vi "D-O Module (Main) 2nd.vi"(7 "Name of Parent Panel":string="Main.vi", 9 "New Center Coords":T1={"Horizontal"=470, "Vertical"=200}, 10 "Config":variant, 11 "Main UI Message Queue":refnum<queue>) -> ()   [LabVIEW 2018, in "D-O Module.lvlib"]
uses:
  D-O Module.lvlib
  support/Message Queue/Message Queue.lvlib
  support/Support Library.lvlib
  support/Message Queue/Enqueue Message (Single).vi
  support/Command Log VIs/Command Logging.lvlib
  controls/UI State.ctl
  Sequencing/Squence Update Cluster.ctl
  Sequencing/Sequencing Library.lvlib
  Measure Instrument/State Enum.ctl
  Measure Instrument/Feed Module Engine.lvlib
  support/User Event - Stop/User Event - Stop.lvlib
  D-O Settings Dialog.vi
  <vilib>/Utility/error.llb/Error Cluster From Error Code.vi
  <vilib>/ErrorRing/Error Ring.xnode
  D-O Module Display.ctl
  VICI Electronic Actuator/VICI Electronic Actuator Settings.ctl
  DIO Valve/VICI Electronic Actuator.lvlib
  D-O Device Settings Cluster.ctl
  D-O Module Settings Cluster.ctl
  Valve Clusters.ctl
  <vilib>/Utility/miscctls.llb/LVPoint32TypeDef.ctl
  D-O Module Config Cluster.ctl
  D-O Module State Cluster.ctl
  controls/UI Data.ctl
  Measure Instrument/D-O Module Engine.lvlib
  support/Message Queue/Message Cluster.ctl
panel:
  out "Sequence Started":bool
  out "ScanCode":i16
  in  "Settings Button":bool
  in  "Exit":bool
  out "Ring":u16(ring)=2
  out "Status":string
  out "Log File path":path
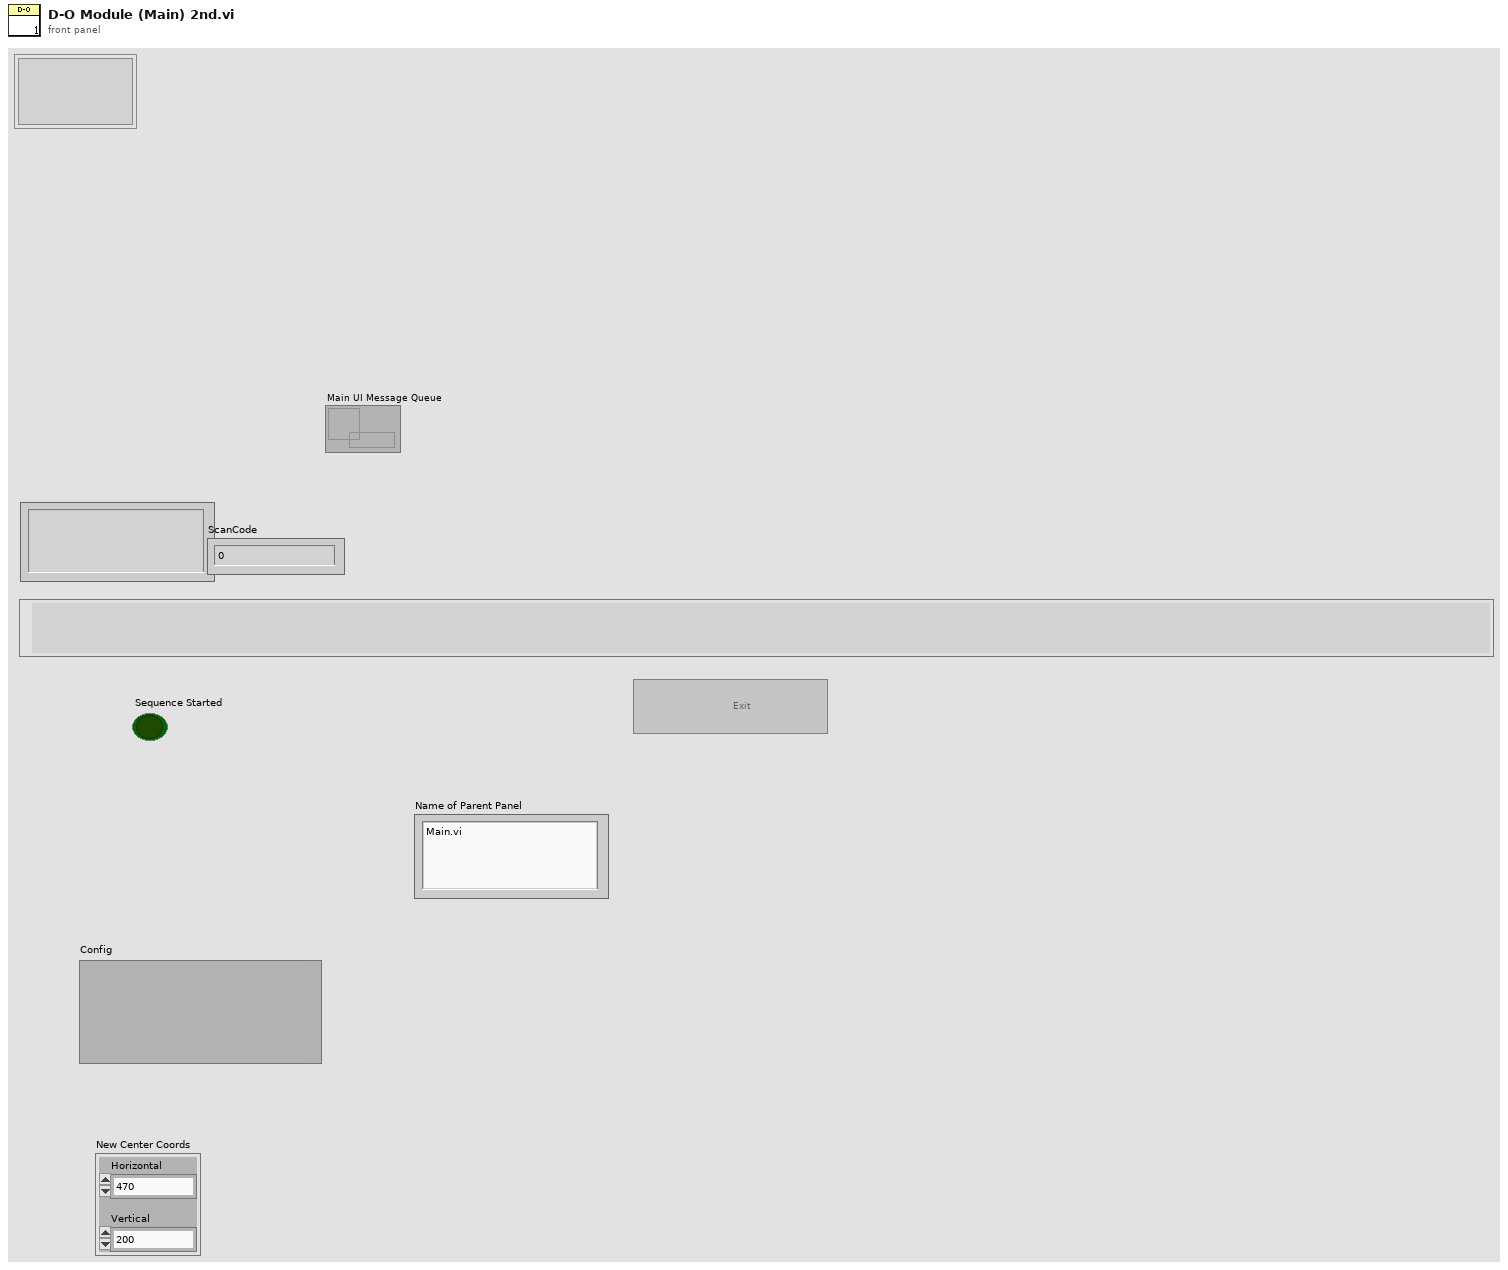
[diagram p1: front panel]
types:
  T1 = typedef "LVPoint32TypeDef.ctl" = cluster{"Horizontal":i32, "Vertical":i32}
  T2 = typedef "UI Data.ctl" = cluster{"Start Ref":refnum<vi>, "Trigger Ref":refnum<vi>, "Stop Ref":refnum<vi>, "Settings Ref":refnum<vi>, "Status Ref":refnum<vi>, "Exit Ref":refnum<vi>, "Data Ref":refnum<vi>}
  T3 = typedef "D-O Module.lvlib/D-O Module State Cluster.ctl" = cluster{"D-O Module Config":T4, "State":T9, "Start Time":timestamp, "Current Time":timestamp, "First Iteration":bool, "Data":cluster{"Valve State":T6}, "Process Name":string, "Queue Name":string, "Program On?":bool}
  T4 = typedef "D-O Module.lvlib/D-O Module Config Cluster.ctl" = cluster{"GUID":string, "Drop Coords":T1, "Process Name":string, "Queue Name":string, "Settings":T5, "Load Count":i32}
  T5 = typedef "D-O Module.lvlib/Valve Clusters.ctl" = cluster{"Valve Settings":T6, "Valve Type":enum16{"Default", "Digital Output Valve", "VICI Electronic Actuator"}, "Time On (Sec)":dbl, "Time Off (Sec)":dbl, "Run?":bool}
  T6 = typedef "D-O Module.lvlib/D-O Module Settings Cluster.ctl" = cluster{"D-O Settings":T7, "VICI Electronic Actuator":T8}
  T7 = typedef "D-O Module.lvlib/D-O Device Settings Cluster.ctl" = cluster{"DAQmx Task Name":refnum<k21>, "Output Channel":u16, "Output Channel Names":string[]}
  T8 = typedef "VICI Electronic Actuator.lvlib/VICI Electronic Actuator Settings.ctl" = cluster{"VISA resource name":refnum<visa-resource-name>, "Mode":enum16{"Two Positions With Stops", "Two Positions Without Stops", "Mutiposition"}, "Simulated":bool}
  T9 = typedef "Feed Module.lvlib/Feed Module Engine.lvlib/State Enum.ctl" = enum16{"Measuring", "Idle", "Paused"}
  T10 = typedef "UI State.ctl" = enum16{"Idle", "Acquiring and Logging", "Waiting for Exit", "Waiting for Exit (Acq Stopped)", "Waiting for Exit (Log Stopped)", "Waiting for Stop", "Waiting for Stop (Acq Stopped)", "Waiting for Stop (Log Stopped)"}
  T11 = typedef "D-O Module.lvlib/All Message Queues.ctl" = cluster{"Engine":refnum<queue>, "D-O UI":refnum<queue>, "D-O Engine":refnum<queue>, "D-O Display":refnum<queue>}
  T12 = typedef "Sequencing Library.lvlib/Squence Update Cluster.ctl" = cluster{"Auto?":bool, "Manual Entry":dbl, "Setpoint":dbl}
  T13 = enum8{"Enabled", "Disabled", "Disabled and Grayed Out"}
  T14 = typedef "D-O Module.lvlib/D-O Module Display.ctl" = cluster{"D-O State ":u16, "Cycle Period":dbl}
  T15 = cluster{"Shift":bool, "Ctrl":bool, "Alt":bool, "Cmd":bool, "Opt":bool}
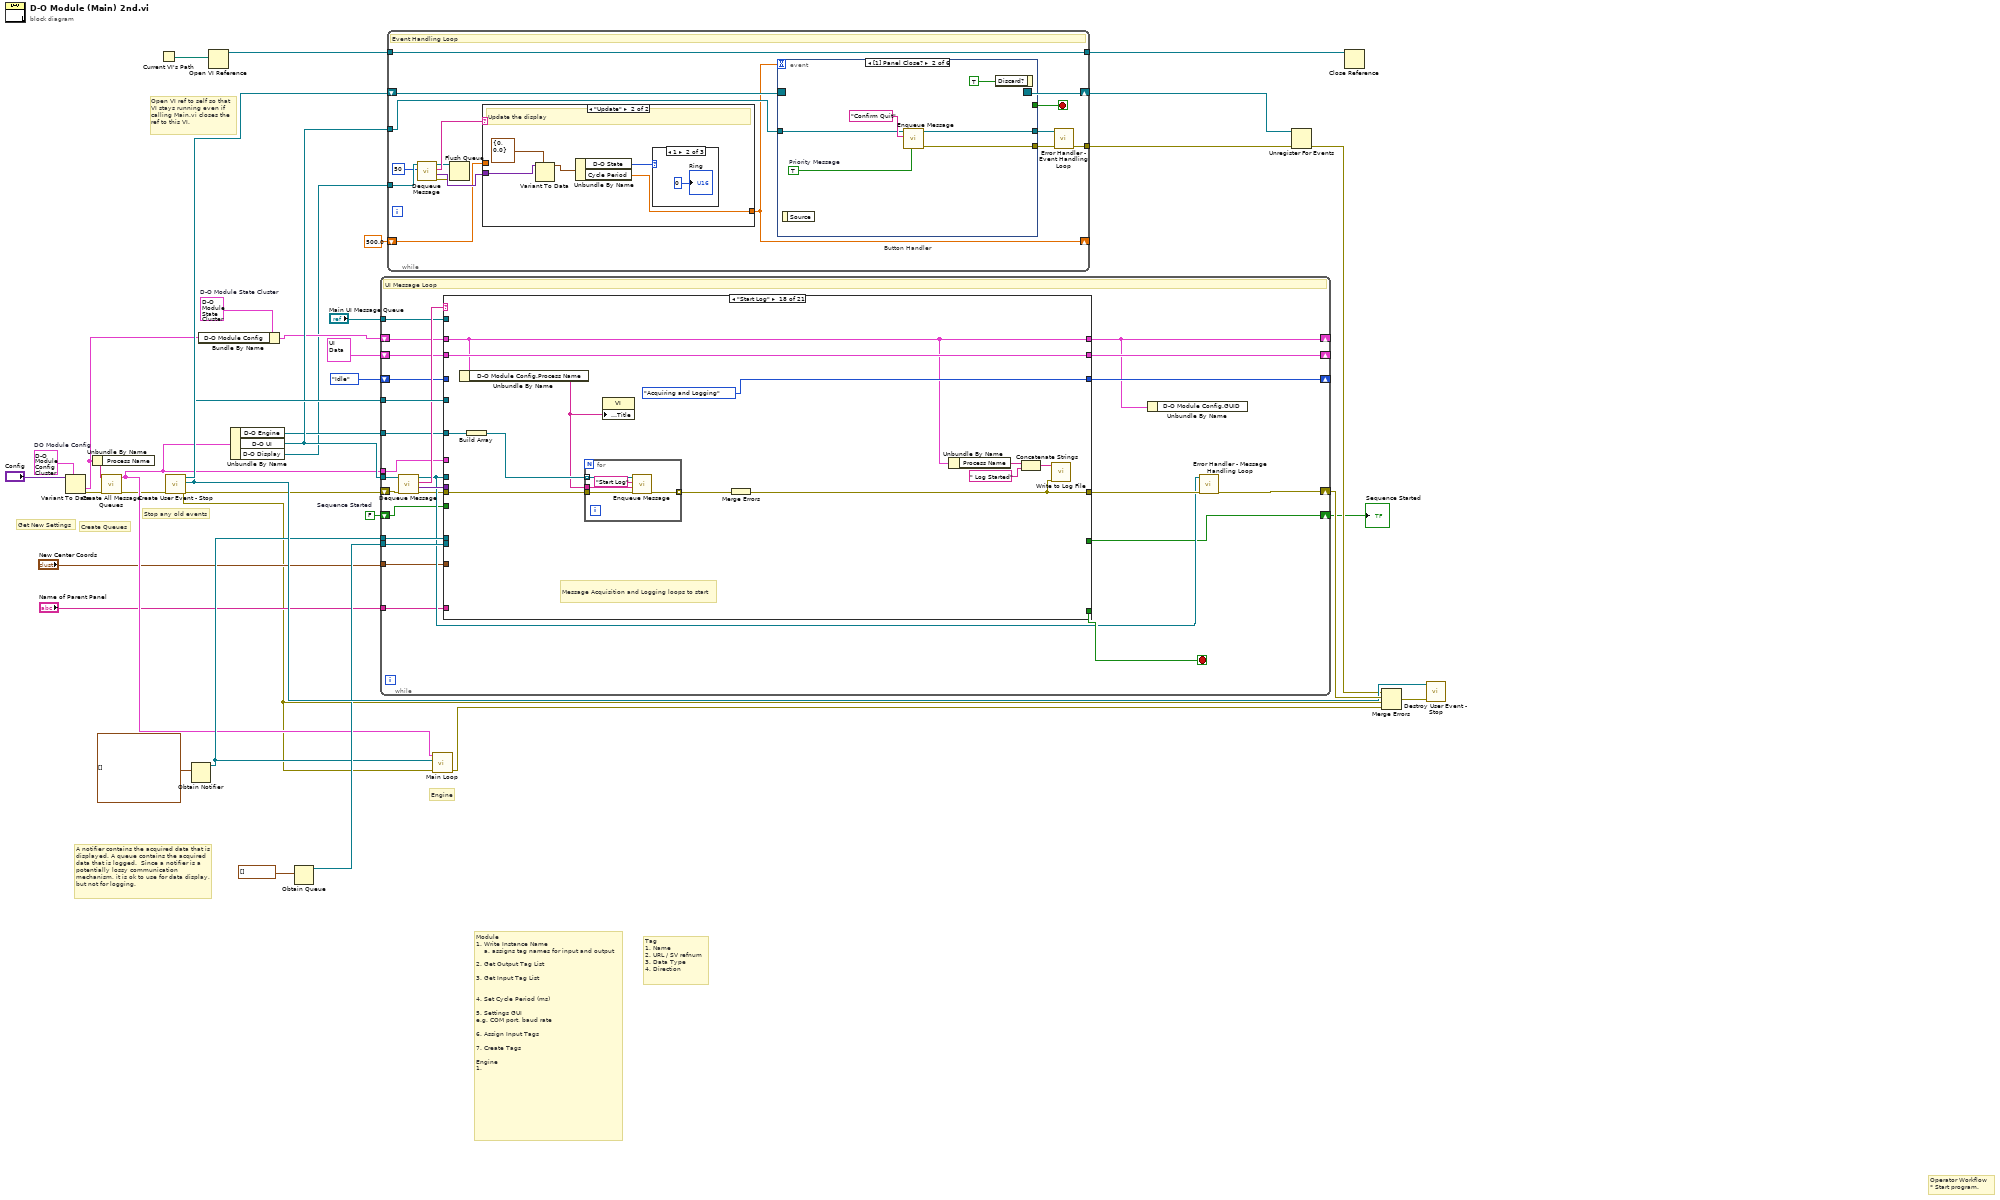
[diagram p0: block diagram]
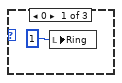
[diagram p3: hidden frame]
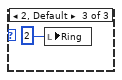
[diagram p4: hidden frame]
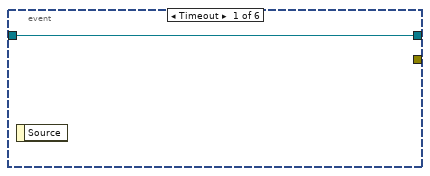
[diagram p5: hidden frame]
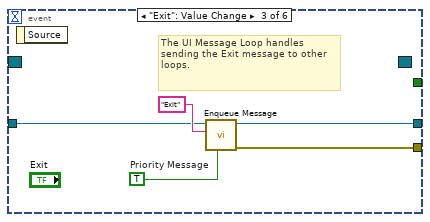
[diagram p6: hidden frame]
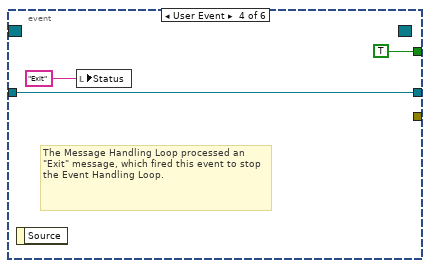
[diagram p7: hidden frame]
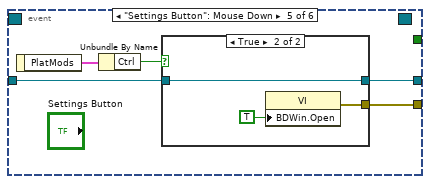
[diagram p8: hidden frame]
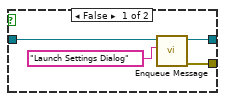
[diagram p9: hidden frame]
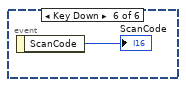
[diagram p10: hidden frame]
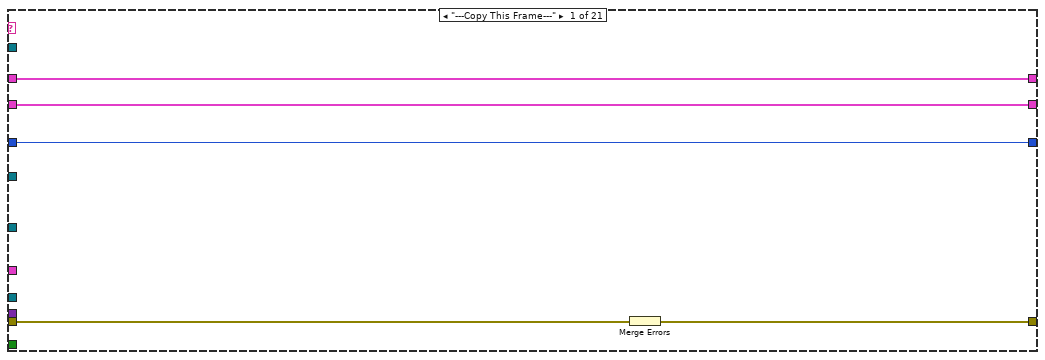
[diagram p11: hidden frame]
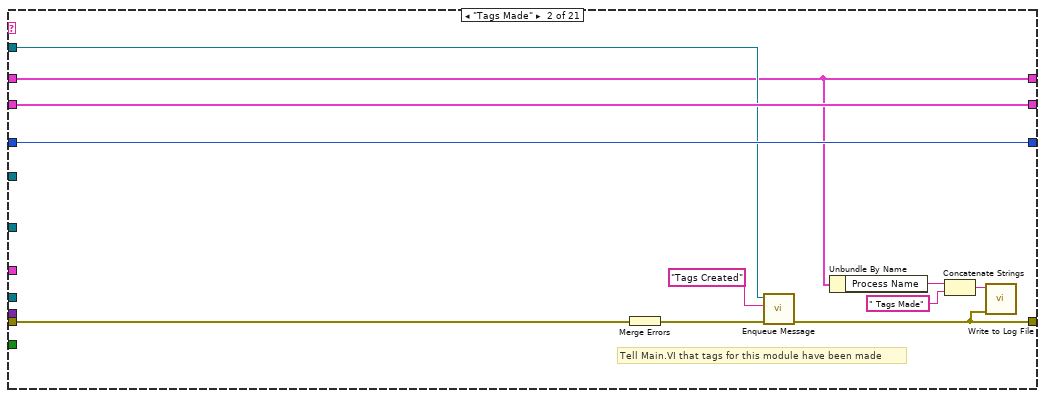
[diagram p12: hidden frame]
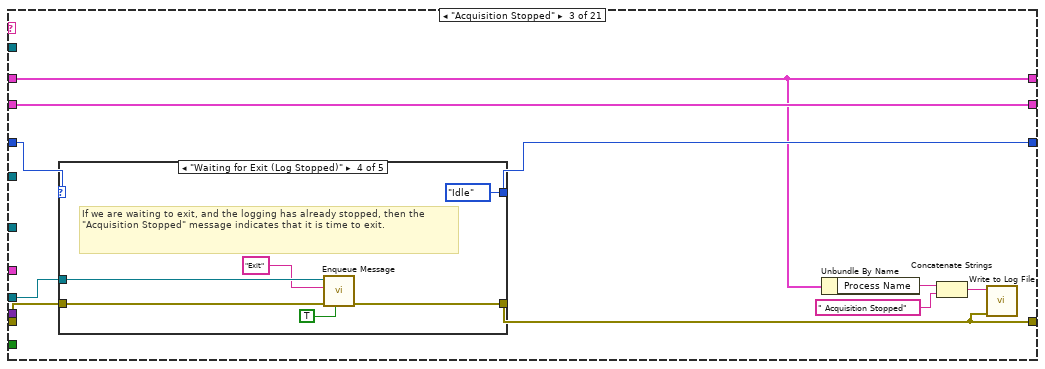
[diagram p13: hidden frame]
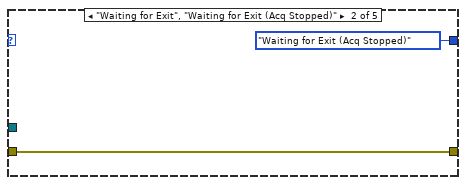
[diagram p15: hidden frame]
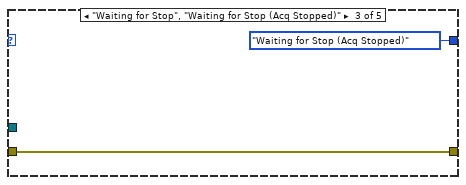
[diagram p16: hidden frame]
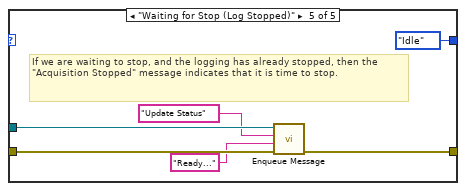
[diagram p17: hidden frame]
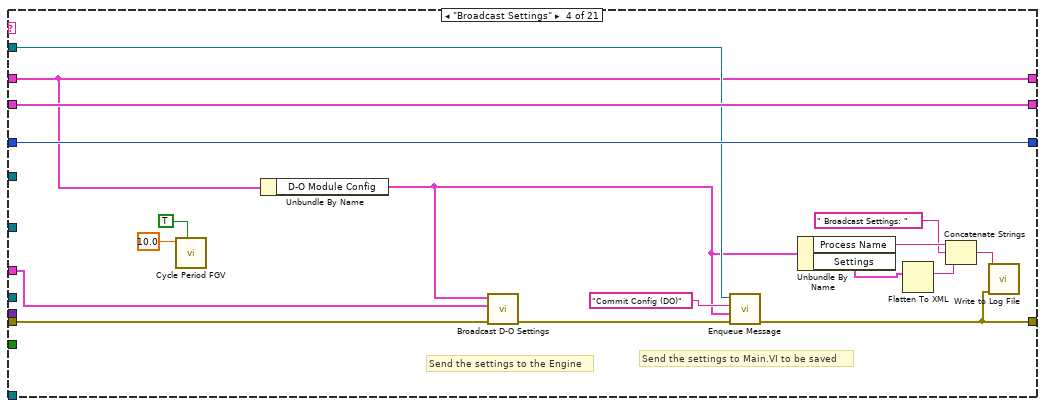
[diagram p18: hidden frame]
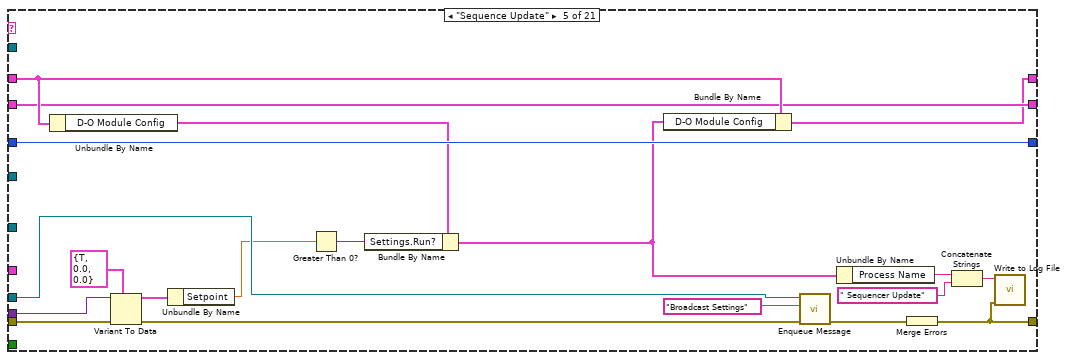
[diagram p19: hidden frame]
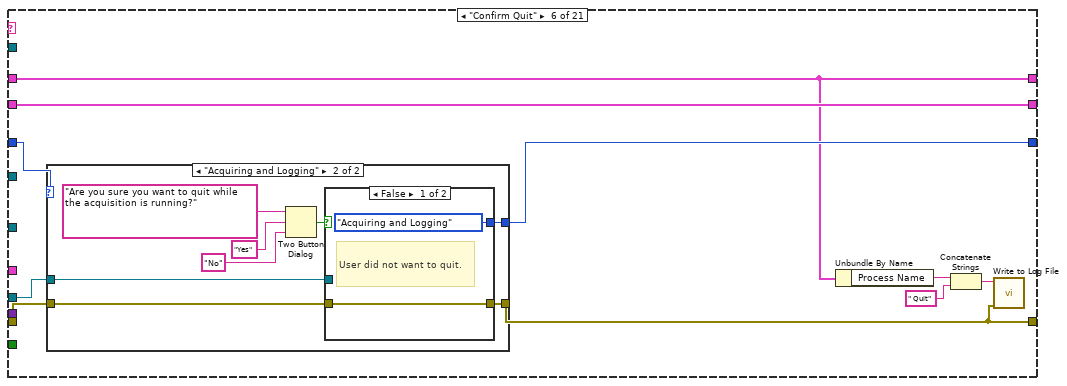
[diagram p20: hidden frame]
diagram:
  w15 = T3 {"D-O Module Config"={"GUID"="", "Drop Coords"={"Horizontal"=0, "Vertical"=0}, "Process Name"="", "Queue Name"="", "Settings"={"Valve Settings"={"D-O Settings"={"DAQmx Task Name"="", "Output Channel"=0, "Output Channel Names"=[]}, "VICI Electronic Actuator"={"VISA resource name"="", "Mode"=enum."Two Positions With Stops", "Simulated"=FALSE}}, "Valve Type"=enum."Digital Output Valve", "Time On (Sec)"=0.0, "Time Off (Sec)"=0.0, "Run?"=FALSE}, "Load Count"=0}, "State"=enum."Idle", "Start Time"=timestamp(0 s since 1904-01-01), "Current Time"=timestamp(0 s since 1904-01-01), "First Iteration"=FALSE, "Data"={"Valve State"={"D-O Settings"={"DAQmx Task Name"="", "Output Channel"=0, "Output Channel Names"=[]}, "VICI Electronic Actuator"={"VISA resource name"="", "Mode"=enum."Two Positions With Stops", "Simulated"=FALSE}}}, "Process Name"="", "Queue Name"="", "Program On?"=FALSE}  # D-O Module State Cluster
  w8 = FALSE  # Sequence Started
  w7 = T4 {"GUID"="", "Drop Coords"={"Horizontal"=0, "Vertical"=0}, "Process Name"="", "Queue Name"="", "Settings"={"Valve Settings"={"D-O Settings"={"DAQmx Task Name"="", "Output Channel"=0, "Output Channel Names"=[]}, "VICI Electronic Actuator"={"VISA resource name"="", "Mode"=enum."Two Positions With Stops", "Simulated"=FALSE}}, "Valve Type"=enum."Default", "Time On (Sec)"=0.0, "Time Off (Sec)"=0.0, "Run?"=FALSE}, "Load Count"=0}  # DO Module Config
  # "Stop any old events"
  # "Create Queues"
  # "Get New Settings"
  # "Open VI ref to self so that\nVI stays running even if\ncalling Main.vi closes the\nref to this VI."
  # "Engine"
  # "Operator Workflow\n* Start program."
  # "Module \n1. Write Instance Name\n    a. assigns tag names for input and output\n\n2. Get Output Tag List\n\n3. Get Input Tag List\n\n\n4. Set Cycle Period (ms)\n\n5. Settings GUI\ne.g. COM port, baud rate\n\n6. Assign Input Tags\n\n7. Create Tags\n\nEngine\n1."
  # "Tag\n1. Name\n2. URL / SV refnum\n3. Data Type\n4. Direction"
  # "A notifier contains the acquired data that is displayed. A queue contains the acquired data that is logged.  Since a notifier is a potentially lossy communication mechanism, it is ok to use for data display, but not for logging."
  n1 = Variant To Data(type=w7, Variant="Config") -> (data=w6:T4, error out=w5:errorcluster)  [unwired: 1 in]
  n2 = Unbundle By Name(w6) -> ("Process Name"=w2:string)
  n3 = call "Create All Message Queues.vi"("error in (no error)"=w5, "Process Name"=w2) -> ("error out"=w4:errorcluster, "Message Queues"=w12:T11)  [unwired: 8 in]
  n4 = Current VI's Path() -> (path=w18:path)
  n5 = call "Create User Event - Stop.vi"("error in (no error)"=w4) -> ("error out"=w3:errorcluster, "User Event - Stop"=w32:refnum<user-event>, "Stop Event Registration Refnum"=w33:refnum<event-registration>)  [unwired: 8 in]
  n6 = Obtain Notifier(notification data type=waveform(dbl)[] []) -> (notifier out=w21:refnum<notifier>)  [unwired: 3 in, 2 out]
  n7 = Bundle By Name(cluster=w15, "D-O Module Config"=w6) -> (w17:T3)
  n8 = Open VI Reference(vi path=w18) -> (vi reference=w19:refnum<vi>)  [unwired: 5 in, 1 out]
  n9 = Unbundle By Name(w12) -> ("D-O Engine"=w24:refnum<queue>, "D-O UI"=w28:refnum<queue>, "D-O Display"=w14:refnum<queue>)
  n10 = Obtain Queue(element data type=waveform(dbl)[] []) -> (queue out=w23:refnum<queue>)  [unwired: 4 in, 2 out]
  n11 = while {
    tunnel: w28 -> [w56]
    tunnel: w32 -> [w60]
    shift-right: [w50] -> w36
    shift-left: w3 -> [w59]
    shift-right: [w37] -> _
    shift-left: w17 -> [w44]
    shift-right: [w54] -> _
    shift-left: T2 {"Start Ref"=refnum, "Trigger Ref"=refnum, "Stop Ref"=refnum, "Settings Ref"=refnum, "Status Ref"=refnum, "Exit Ref"=refnum, "Data Ref"=refnum} ("Measurement UI Controls") -> [w55]
    tunnel: w21 -> [w53]
    tunnel: w23 -> [w52]
    shift-right: [w47] -> _
    shift-left: UI_State."Idle" ("UI State") -> [w48]
    tunnel: w24 -> [w46]
    tunnel: "Main UI Message Queue" -> [w43]
    tunnel: w12 -> [w42]
    tunnel: "New Center Coords" -> [w41]
    tunnel: "Name of Parent Panel" -> [w40]
    shift-right: [w39] -> w9
    shift-left: w8 -> [w38]
    stop <- w61 stop-if-true
    # "UI Message Loop"
    n12 = call "Dequeue Message.vi"("error in (no error)"=w59, "Message Queue"=w56) -> ("error out"=w45:errorcluster, "Message Data"=w57:variant, "Message"=w58:string, "dup Message Queue"=w49:refnum<queue>)  [unwired: 6 in]
    n13 = case "Message Cases" shown="\"Start Log\"" w58 {
      selector: w58 -> [_ _ _ _ _ _ _ _ _ _ _ _ _ _ _ _ _ _ _ _ w486]
      tunnel: w49 -> [_ _ w83 _ w138 w150 _ w208 w223 w250 _ w284 w303 w309 w345 w377 _ _ w442 _ _]
      tunnel: w45 -> [w66 w77 w84 w119 w136 w149 w176 w189 w227 w254 w269 w279 w300 w311 w343 w376 w403 w424 w444 w477 _]
      tunnel: [w65 w71 w82 w112 w124 w144 w177 w183 w217 w229 w269 w274 w295 w310 w334 w365 w407 w422 w439 w478 w489] -> w51
      tunnel: [_ _ _ _ _ _ _ _ _ TRUE _ _ _ _ _ _ _ _ _ _ _] -> w61
      tunnel: w57 -> [_ _ _ _ w139 _ w179 _ w226 w238 _ _ _ _ _ _ _ _ _ w476 _]
      tunnel: w60 -> [_ _ _ _ _ _ _ _ _ w253 _ _ _ _ _ _ _ _ _ _ _]
      tunnel: w44 -> [w62 w67 w78 w116 w141 w143 w174 w187 w214 w230 w260 w270 w302 w308 w339 w372 w401 w418 w446 w467 w484]
      tunnel: w55 -> [w64 w76 w87 w122 w140 w152 w181 w205 w228 w251 w268 w280 w307 w314 w340 w373 w406 w429 w462 w473 w491]
      tunnel: [w64 w76 w87 w122 w140 w152 w181 w205 w228 w251 w267 w280 w307 w314 w340 w373 w406 w429 w462 w473 w491] -> w54
      tunnel: w53 -> [_ _ _ _ _ _ _ _ _ w249 _ _ _ _ _ _ _ _ _ _ _]
      tunnel: w52 -> [_ _ _ _ _ _ _ _ _ w245 _ _ _ _ _ _ _ _ _ _ _]
      tunnel: w48 -> [w63 w75 w86 w121 w142 w151 w175 w194 w218 _ _ _ w306 w313 _ _ _ _ w451 w468 w490]
      tunnel: [w63 w75 w85 w121 w142 w148 w175 w195 w218 UI_State."Idle" ("UI State") UI_State."Idle" ("UI State") UI_State."Idle" ("UI State") w306 w312 UI_State."Acquiring and Logging" ("UI State") UI_State."Acquiring and Logging" ("UI State") UI_State."Acquiring and Logging" ("UI State") UI_State."Acquiring and Logging" ("UI State") w452 w468 w490] -> w47
      tunnel: w46 -> [_ _ _ _ _ _ _ w193 _ w237 _ _ _ _ _ _ w404 w427 w450 _ _]
      tunnel: w43 -> [_ w72 _ w118 _ _ _ _ _ w239 _ _ _ _ _ _ _ _ _ _ _]
      tunnel: [w62 w67 w78 w116 w137 w143 w174 w182 w214 w230 w260 w270 w291 w308 w333 w362 w401 w418 w435 w467 w484] -> w37
      tunnel: w42 -> [_ _ _ w114 _ _ _ _ _ _ _ _ w297 _ _ _ _ _ _ _ _]
      tunnel: w41 -> [_ _ _ _ _ _ _ _ _ _ _ w277 _ _ _ _ _ _ _ _ _]
      tunnel: w40 -> [_ _ _ _ _ _ _ _ _ _ _ w276 _ _ _ _ _ _ _ _ _]
      tunnel: [_ _ _ _ _ _ _ _ _ _ _ _ _ _ _ w370 _ _ _ _ _] -> w39
      tunnel: w38 -> [_ _ _ _ _ _ _ _ _ _ _ _ _ _ _ w366 _ _ _ _ _]
      frame "---Copy This Frame---" {
        # "Duplicate this frame when creating new messages.  Change this comment in the duplicated frame to describe this message."
        n14 = Merge Errors(w66) -> (w65:errorcluster)
      }
      frame "Tags Made" {
        # "Tell Main.VI that tags for this module have been made"
        # "Duplicate this frame when creating new messages.  Change this comment in the duplicated frame to describe this message."
        n15 = Merge Errors(w77) -> (w73:errorcluster)
        n16 = call-poly "Enqueue Message.vi"("error in (no error)"=w73, "Message"="Tags Created", "Message Queue"=w72) -> ("error out"=w71:errorcluster)  [unwired: 7 in, 1 out]
        n17 = Unbundle By Name(w67) -> ("Process Name"=w70:string)
        n18 = Concatenate Strings(w70, " Tags Made" ("text")) -> (w68:string)
        n19 = call "Write to Log File.vi"("error in"=w71, "text"=w68) -> ()  [unwired: 9 in, 1 out]
      }
      frame "Acquisition Stopped" {
        # "Logic for determining what action to take when the acquisition has stopped."
        n20 = case shown="\"Waiting for Exit (Log Stopped)\"" w86 {
          selector: w86 -> [w89 _ _ _ _]
          tunnel: [w89 UI_State."Waiting for Exit (Acq Stopped)" ("UI State") UI_State."Waiting for Stop (Acq Stopped)" ("UI State") UI_State."Idle" ("UI State") UI_State."Idle" ("UI State")] -> w85
          tunnel: w84 -> [w88 w90 w92 w98 w104]
          tunnel: [w88 w90 w92 w97 w103] -> w82
          tunnel: w83 -> [_ _ _ w96 w102]
          frame Default {
          }
          frame "Waiting for Exit", "Waiting for Exit (Acq Stopped)" {
          }
          frame "Waiting for Stop", "Waiting for Stop (Acq Stopped)" {
          }
          frame "Waiting for Exit (Log Stopped)" {
            # "If we are waiting to exit, and the logging has already stopped, then the \"Acquisition Stopped\" message indicates that it is time to exit."
            n21 = call-poly "Enqueue Message.vi"("Priority Message? (F)"=TRUE, "error in (no error)"=w98, "Message"="Exit", "Message Queue"=w96) -> ("error out"=w97:errorcluster)  [unwired: 6 in, 1 out]
          }
          frame "Waiting for Stop (Log Stopped)" {
            # "If we are waiting to stop, and the logging has already stopped, then the \"Acquisition Stopped\" message indicates that it is time to stop."
            n22 = call-poly "Enqueue Message.vi"("error in (no error)"=w104, "Message Data"="Ready..." ("Message"), "Message"="Update Status", "Message Queue"=w102) -> ("error out"=w103:errorcluster)  [unwired: 6 in, 1 out]
          }
        }
        n23 = Unbundle By Name(w78) -> ("Process Name"=w81:string)
        n24 = Concatenate Strings(w81, " Acquisition Stopped" ("text")) -> (w79:string)
        n25 = call "Write to Log File.vi"("error in"=w82, "text"=w79) -> ()  [unwired: 9 in, 1 out]
      }
      frame "Broadcast Settings" {
        # "Send the settings to Main.VI to be saved"
        # "Send the settings to the Engine"
        # "Send the 'Update Settings' message to the Logging and Acquisition message loops."
        n26 = call "Cycle Period FGV.vi"("Write"=TRUE, "Cycle Period In (ms)"=10.0) -> ()  [unwired: 8 in, 2 out]
        n27 = Unbundle By Name(w116) -> ("D-O Module Config"=w108:T4)
        n28 = call "Broadcast D-O Settings.vi"("error in (no error)"=w119, "Message Queues"=w114, "D-O Module Config"=w108) -> ("error out"=w117:errorcluster)  [unwired: 8 in]
        n29 = call-poly "Enqueue Message.vi"("error in (no error)"=w117, "Message Data"=w108, "Message"="Commit Config (DO)", "Message Queue"=w118) -> ("error out"=w112:errorcluster)  [unwired: 6 in, 1 out]
        n30 = Unbundle By Name(w108) -> ("Process Name"=w111:string, "Settings"=w106:T5)
        n31 = Flatten To XML(anything=w106) -> (xml string=w107:string)
        n32 = Concatenate Strings(w111, " Broadcast Settings: " ("text"), w107) -> (w109:string)
        n33 = call "Write to Log File.vi"("error in"=w112, "text"=w109) -> ()  [unwired: 9 in, 1 out]
      }
      frame "Sequence Update" {
        n34 = Unbundle By Name(w141) -> ("D-O Module Config"=w135:T4)
        n35 = Variant To Data(error in=w136, type=T12 {"Auto?"=TRUE, "Manual Entry"=0.0, "Setpoint"=0.0} ("Cluster"), Variant=w139) -> (data=w133:T12, error out=w130:errorcluster)
        n36 = Unbundle By Name(w133) -> ("Setpoint"=w128:dbl)
        n37 = Greater Than 0?(x=w128) -> (x > 0?=w129:bool)
        n38 = Bundle By Name(cluster=w135, "Settings.Run?"=w129) -> (w123:T4)
        n39 = Bundle By Name(cluster=w141, "D-O Module Config"=w123) -> (w137:T3)
        n40 = call-poly "Enqueue Message.vi"("error in (no error)"=w130, "Message"="Broadcast Settings", "Message Queue"=w138) -> ("error out"=w132:errorcluster)  [unwired: 7 in, 1 out]
        n41 = Unbundle By Name(w123) -> ("Process Name"=w127:string)
        n42 = Merge Errors(w132) -> (w124:errorcluster)
        n43 = Concatenate Strings(w127, " Sequencer Update" ("text")) -> (w125:string)
        n44 = call "Write to Log File.vi"("error in"=w124, "text"=w125) -> ()  [unwired: 9 in, 1 out]
      }
      frame "Confirm Quit" {
        # "Confirm Quit - Message that can confirm whether or not the user wants to exit the application."
        n45 = case shown="\"Acquiring and Logging\"" w151 {
          tunnel: w150 -> [w157 w163]
          tunnel: w149 -> [w156 w161]
          tunnel: [w153 w160] -> w144
          tunnel: [UI_State."Idle" ("UI State") w159] -> w148
          frame Default {
            # "If 'Confirm Quit' comes in while the system is idle, there is no need for a confirmation message."
            n46 = call-poly "Enqueue Message.vi"("Priority Message? (F)"=TRUE, "error in (no error)"=w156, "Message"="Exit", "Message Queue"=w157) -> ("error out"=w153:errorcluster)  [unwired: 6 in, 1 out]
          }
          frame "Acquiring and Logging" {
            n47 = Two Button Dialog(message="Are you sure you want to quit while the acquisition is running?" ("Confirm Quit Message"), 1:"No" ("No"), 2:"Yes" ("Yes")) -> (T button?=w162:bool)
            n48 = case shown="False" w162 {
              tunnel: w163 -> [_ w173]
              tunnel: w161 -> [w167 w172]
              tunnel: [w167 w171] -> w160
              tunnel: [UI_State."Acquiring and Logging" ("UI State") UI_State."Waiting for Exit" ("UI State")] -> w159
              frame False {
                # "User did not want to quit."
              }
              frame True {
                n49 = call-poly "Enqueue Message.vi"("error in (no error)"=w172, "Message"="Stop", "Message Queue"=w173) -> ("error out"=w171:errorcluster)  [unwired: 7 in, 1 out]
              }
            }
          }
        }
        n50 = Unbundle By Name(w143) -> ("Process Name"=w147:string)
        n51 = Concatenate Strings(w147, " Quit" ("text")) -> (w145:string)
        n52 = call "Write to Log File.vi"("error in"=w144, "text"=w145) -> ()  [unwired: 9 in, 1 out]
      }
      frame "Display Log File Path" {
        n53 = Variant To Data(error in=w176, type=path "", Variant=w179) -> (data=→"Log File path":path, error out=w177:errorcluster)
      }
      frame "E-Stop" {
        # "Pause the DO when E-Stop is sent"
        # "Message Acquisition and Logging loops to stop"
        # "Enable: Start, Exit, Settings\nDisable: Stop"
        # "Stop the pumps."
        n54 = Unbundle By Name(w205) -> ("Trigger Ref"=w196:refnum<vi>, "Stop Ref"=w197:refnum<vi>, "Start Ref"=w200:refnum<vi>, "Exit Ref"=w199:refnum<vi>, "Settings Ref"=w198:refnum<vi>)
        n55 = call-poly "Enqueue Message.vi"("error in (no error)"=w189, "Message Data"="Ready..." ("Ready..."), "Message"="Update Status", "Message Queue"=w208) -> ("error out"=w191:errorcluster)  [unwired: 6 in, 1 out]
        n56 = Build Array(w200, w199, w198) -> (w203:refnum<vi>[])
        n57 = Build Array(w196, w197) -> (w202:refnum<vi>[])
        n58 = call-poly "Enqueue Message.vi"("error in (no error)"=w191, "Message"="Pause", "Message Queue"=w193) -> ("error out"=w190:errorcluster)  [unwired: 7 in, 1 out]
        n59 = call "Set Enable State on Multiple Controls.vi"("Enable?"=FALSE, "Controls"=w202) -> ()  [unwired: 10 in]
        n60 = call "Set Enable State on Multiple Controls.vi"("Enable?"=TRUE, "Controls"=w203) -> ()  [unwired: 10 in]
        n61 = case shown="Default" w194 {
          selector: w194 -> [_ w210]
          tunnel: [UI_State."Waiting for Stop" ("UI State") w210] -> w195
          frame Default {
          }
          frame "Waiting for Exit" {
          }
        }
        n62 = Merge Errors(w190) -> (w183:errorcluster)
        n63 = Bundle By Name(cluster=w187, "State"=State_Enum."Idle") -> (w182:T3)
        n64 = Unbundle By Name(w182) -> ("Process Name"=w186:string)
        n65 = Concatenate Strings(w186, " E-STOP" ("text")) -> (w184:string)
        n66 = call "Write to Log File.vi"("error in"=w183, "text"=w184) -> ()  [unwired: 9 in, 1 out]
      }
      frame "Error" {
        # "Error - Check the error message data and respond accordingly. This message is sent by the \"Error Handler\" VIs at the end of each loop in this application."
        n67 = Variant To Data(error in=w227, type=errorcluster {"status"=FALSE, "code"=0, "source"=""} ("error out"), Variant=w226) -> (data=w224:errorcluster, error out=w220:errorcluster)
        n68 = call <vilib>:"Simple Error Handler.vi"("error in (no error)"=w224) -> ()  [unwired: 4 in, 5 out]
        n69 = call-poly "Enqueue Message.vi"("Priority Message? (F)"=TRUE, "Message"="Exit", "Message Queue"=w223) -> ("error out"=w219:errorcluster)  [unwired: 7 in, 1 out]
        n70 = Merge Errors(w219, w220) -> (w217:errorcluster)
        n71 = Unbundle By Name(w214) -> ("Process Name"=w216:string)
        n72 = call <vilib>:"General Error Handler.vi"("error in (no error)"=w217) -> ("message"=w212:string, "error out"=w211:errorcluster)  [unwired: 10 in, 3 out]
        n73 = Concatenate Strings(w216, " Error: " ("text"), w212) -> (w215:string)
        n74 = call "Write to Log File.vi"("error in"=w211, "text"=w215) -> ()  [unwired: 9 in, 1 out]
      }
      frame "Exit" {
        w242 = TRUE  # Delete Module?
        # "Stop DO Engine then Close it"
        # "Don't check the error outs. The acquisition and logging queues may have already been released."
        # "Close references owned by the Main VI."
        # "Stop the VI"
        # "Exit - Fire the User Event to stop the Event Handling Loop.  Also send Exit messages to the Acquisition and Logging loops."
        n75 = Release Queue(queue=w250, error in (no error)=w254) -> (error out=w248:errorcluster)  [unwired: 1 in, 2 out]
        n76 = call "Fire User Event - Stop.vi"("User Event - Stop"=w253) -> ("error out"=w252:errorcluster)  [unwired: 10 in]
        n77 = Release Notifier(notifier=w249, error in (no error)=w248) -> (error out=w247:errorcluster)  [unwired: 1 in, 2 out]
        n78 = Release Queue(queue=w245, error in (no error)=w247) -> (error out=w246:errorcluster)  [unwired: 1 in, 2 out]
        n79 = call-poly "Enqueue Message.vi"("Message"="Stop", "Message Queue"=w237) -> ("dup Message Queue"=w235:refnum<queue>)  [unwired: 8 in, 1 out]
        n80 = Variant To Data(type=w242, Variant=w238) -> (data=w241:bool, error out=w243:errorcluster)  [unwired: 1 in]
        n81 = Select(t=w242, s=w243, f=w241) -> (s? t:f=w240:bool)
        n82 = call-poly "Enqueue Message.vi"("Message"="Exit", "Message Queue"=w235) -> ()  [unwired: 8 in, 2 out]
        n83 = case "Don't enqueue Delete Module if opening campaign because it\nwill already have been deleted and new config loaded and we create\na race condition." shown="True" w240 {
          tunnel: w239 -> [_ w258]
          tunnel: w230 -> [_ w257]
          frame False {
          }
          frame True {
            n84 = Unbundle By Name(w257) -> ("D-O Module Config.GUID"=w256:string)
            n85 = call-poly "Enqueue Message.vi"("Message Data"=w256, "Message"="Delete Module", "Message Queue"=w258) -> ()  [unwired: 7 in, 2 out]
          }
        }
        n86 = Merge Errors(w252, w246) -> (w229:errorcluster)
        n87 = Unbundle By Name(w230) -> ("Process Name"=w233:string)
        n88 = Concatenate Strings(w233, " Exit" ("text")) -> (w231:string)
        n89 = call "Write to Log File.vi"("error in"=w229, "text"=w231) -> ()  [unwired: 9 in, 1 out]
      }
      frame "Init UI Refs" {
        # "Enable: Start, Exit, Settings\nDisable: Stop"
        # "Init UI Refs - Store control references for UI controls.  Also enable/disable controls appropriately."
        n90 = property class="VI"("Front Panel.Closeable"=TRUE ("Front Panel Window:Closeable")) -> ()  [unwired: 2 in, 2 out]
        n91 = control-ref of="Status"() -> (w265:refnum<vi>)
        n92 = control-ref of="Exit"() -> (w262:refnum<vi>)
        n93 = Bundle By Name(cluster=w268, "Status Ref"=w265, "Exit Ref"=w262) -> (w267:T2)
        n94 = Build Array(w262) -> (w264:refnum<vi>[])
        n95 = call "Set Enable State on Multiple Controls.vi"("Enable?"=TRUE, "Controls"=w264) -> ()  [unwired: 10 in]
      }
      frame "Initialize" {
        # "Initialize - Get configuration settings, then message the UI to initialize, and broadcast the settings to the other message loops."
        n96 = Unbundle By Name(w270) -> ("Process Name"=w275:string)
        n97 = property class="VI" props=["FP.State"]() -> (reference out=w278:refnum<vi>)  [unwired: 2 in, 2 out]
        n98 = call-poly "Enqueue Message.vi"("error in (no error)"=w279, "Message"="Init UI Refs", "Message Queue"=w284) -> ("error out"=w282:errorcluster, "dup Message Queue"=w283:refnum<queue>)  [unwired: 7 in]
        n99 = call "Make Child and Move.vi"("Process Name"=w275, "Name of Parent Panel"=w276, "New Center Coords"=w277, "VI in"=w278) -> ()  [unwired: 8 in]
        n100 = call-poly "Enqueue Message.vi"("error in (no error)"=w282, "Message"="Broadcast Settings", "Message Queue"=w283) -> ("error out"=w290:errorcluster, "dup Message Queue"=w289:refnum<queue>)  [unwired: 7 in]
        n101 = call-poly "Enqueue Message.vi"("error in (no error)"=w290, "Message Data"="Ready..." ("Ready..."), "Message"="Update Status", "Message Queue"=w289) -> ("error out"=w274:errorcluster)  [unwired: 6 in, 1 out]
        n102 = Unbundle By Name(w270) -> ("Process Name"=w273:string)
        n103 = Concatenate Strings(w273, " Initialize" ("text")) -> (w271:string)
        n104 = call "Write to Log File.vi"("error in"=w274, "text"=w271) -> ()  [unwired: 9 in, 1 out]
      }
      frame "Launch Settings Dialog" {
        # "Keep track of whether the Dialog has been opened."
        # "Launch the Settings Dialog when the user clicks the 'Settings' button."
        n105 = Unbundle By Name(w302) -> ("D-O Module Config.Load Count"=w304:i32)
        n106 = Increment(x=w304) -> (x+1=w305:i32)
        n107 = Bundle By Name(cluster=w302, "D-O Module Config.Load Count"=w305) -> (w298:T3)
        n108 = call-by-ref "?"("error in (no error)"=w300, "Message Queues"=w297, "D-O Module State Cluster In"=w298) -> ("error out"=w296:errorcluster, "D-O Module Config Out"=w299:T4)  [unwired: 7 in, 4 out]
        n109 = Bundle By Name(cluster=w302, "D-O Module Config"=w299) -> (w291:T3)
        n110 = call-poly "Enqueue Message.vi"("error in (no error)"=w296, "Message"="Broadcast Settings", "Message Queue"=w303) -> ("error out"=w295:errorcluster)  [unwired: 7 in, 1 out]
        n111 = Unbundle By Name(w291) -> ("Process Name"=w294:string)
        n112 = Concatenate Strings(w294, "Launch Settings Dialog" ("text")) -> (w292:string)
        n113 = call "Write to Log File.vi"("error in"=w295, "text"=w292) -> ()  [unwired: 9 in, 1 out]
      }
      frame "Logging Stopped" {
        # "Logic for determining what action to take when the logging has stopped."
        n114 = case shown="\"Waiting for Exit (Acq Stopped)\"" w313 {
          selector: w313 -> [w316 _ _ _ _]
          tunnel: [w316 UI_State."Waiting for Exit (Log Stopped)" ("UI State") UI_State."Waiting for Stop (Log Stopped)" ("UI State") UI_State."Idle" ("UI State") UI_State."Idle" ("UI State")] -> w312
          tunnel: w311 -> [w315 w317 w319 w325 w331]
          tunnel: [w315 w317 w319 w324 w330] -> w310
          tunnel: w309 -> [_ _ _ w323 w329]
          frame Default {
          }
          frame "Waiting for Exit", "Waiting for Exit (Log Stopped)" {
          }
          frame "Waiting for Stop", "Waiting for Stop (Log Stopped)" {
          }
          frame "Waiting for Exit (Acq Stopped)" {
            # "If we are waiting to exit, and the acquisition has already stopped, then the \"Logging Stopped\" message indicates that it is time to exit."
            n115 = call-poly "Enqueue Message.vi"("Priority Message? (F)"=TRUE, "error in (no error)"=w325, "Message"="Exit", "Message Queue"=w323) -> ("error out"=w324:errorcluster)  [unwired: 6 in, 1 out]
          }
          frame "Waiting for Stop (Acq Stopped)" {
            # "If we are waiting to stop, and the acquisition has already stopped, then the \"Logging Stopped\" message indicates that it is time to stop."
            n116 = call-poly "Enqueue Message.vi"("error in (no error)"=w331, "Message Data"="Ready..." ("Message"), "Message"="Update Status", "Message Queue"=w329) -> ("error out"=w330:errorcluster)  [unwired: 6 in, 1 out]
          }
        }
      }
      frame "Start" {
        # "Start the loops. In this case we could\n just do a straight start since there is \nonly one loop"
        # "Clear chart"
        # "Message Acquisition and Logging loops to start"
        # "Enable: Stop\nDisable: Start, Exit, Settings"
        # "Start - Enable/Disable buttons appropriately for an acquisition that has started, and update status display."
        n117 = Unbundle By Name(w340) -> ("Trigger Ref"=w351:refnum<vi>, "Stop Ref"=w352:refnum<vi>, "Start Ref"=w355:refnum<vi>, "Exit Ref"=w354:refnum<vi>, "Settings Ref"=w353:refnum<vi>, "Data Ref"=w342:refnum<vi>)
        n118 = property class="WFChart (strict)"(reference=w342, "History Data"=waveform(dbl)[][] []) -> ()  [unwired: 1 in, 2 out]
        n119 = Build Array(w355, w354, w353) -> (w358:refnum<vi>[])
        n120 = Build Array(w351, w352) -> (w357:refnum<vi>[])
        n121 = call-poly "Enqueue Message.vi"("error in (no error)"=w343, "Message"="Broadcast settings", "Message Queue"=w345) -> ("error out"=w346:errorcluster, "dup Message Queue"=w344:refnum<queue>)  [unwired: 7 in]
        n122 = call "Set Enable State on Multiple Controls.vi"("Enable?"=TRUE, "Controls"=w357) -> ()  [unwired: 10 in]
        n123 = call "Set Enable State on Multiple Controls.vi"("Enable?"=FALSE, "Controls"=w358) -> ()  [unwired: 10 in]
        n124 = call-poly "Enqueue Message.vi"("error in (no error)"=w346, "Message"="Start Loops", "Message Queue"=w344) -> ("error out"=w347:errorcluster)  [unwired: 7 in, 1 out]
        n125 = Merge Errors(w347) -> (w334:errorcluster)
        n126 = disable-structure shown="Enabled" {
          disable-tunnel: w339 -> [w360 _]
          frame Disabled {
            n127 = Unbundle By Name(w360) -> ()  [unwired: 1 out]
          }
          frame Enabled {
          }
        }
        n128 = Bundle By Name(cluster=w339, "State"=State_Enum."Measuring") -> (w333:T3)
        n129 = Unbundle By Name(w333) -> ("Process Name"=w337:string)
        n130 = Concatenate Strings(w337, " Start" ("text")) -> (w335:string)
        n131 = call "Write to Log File.vi"("error in"=w334, "text"=w335) -> ()  [unwired: 9 in, 1 out]
      }
      frame "Sequence Start" {
        # "Clear chart"
        # "Message Acquisition and Logging loops to start"
        # "Enable: Stop\nDisable: Start, Exit, Settings"
        # "Start - Enable/Disable buttons appropriately for an acquisition that has started, and update status display."
        n132 = Unbundle By Name(w373) -> ("Trigger Ref"=w380:refnum<vi>, "Stop Ref"=w381:refnum<vi>, "Start Ref"=w384:refnum<vi>, "Exit Ref"=w383:refnum<vi>, "Settings Ref"=w382:refnum<vi>, "Data Ref"=w375:refnum<vi>)
        n133 = property class="WFChart (strict)"(reference=w375, "History Data"=waveform(dbl)[][] []) -> ()  [unwired: 1 in, 2 out]
        n134 = Build Array(w384, w383, w382) -> (w387:refnum<vi>[])
        n135 = Build Array(w380, w381) -> (w386:refnum<vi>[])
        n136 = call-poly "Enqueue Message.vi"("error in (no error)"=w376, "Message"="Broadcast settings", "Message Queue"=w377) -> ("error out"=w369:errorcluster, "dup Message Queue"=w368:refnum<queue>)  [unwired: 7 in]
        n137 = call "Set Enable State on Multiple Controls.vi"("Enable?"=TRUE, "Controls"=w386) -> ()  [unwired: 10 in]
        n138 = call "Set Enable State on Multiple Controls.vi"("Enable?"=FALSE, "Controls"=w387) -> ()  [unwired: 10 in]
        n139 = case shown="False" w366 {
          selector: w366 -> [_ w394]
          tunnel: [w393 w394] -> w370
          tunnel: w369 -> [w392 w395]
          tunnel: w368 -> [w390 _]
          tunnel: [w389 w395] -> w367
          frame False {
            w393 = TRUE  # Sequence Started
            # "Start the loops. In this case we could\n just do a straight start since there is \nonly one loop"
            # "Start the sequence loops"
            n140 = call-poly "Enqueue Message.vi"("error in (no error)"=w392, "Message"="Start Loops", "Message Queue"=w390) -> ("error out"=w389:errorcluster)  [unwired: 7 in, 1 out]
          }
          frame True {
            # "Sequence already started"
          }
        }
        n141 = Merge Errors(w367) -> (w365:errorcluster)
        n142 = Bundle By Name(cluster=w372, "State"=State_Enum."Measuring") -> (w362:T3)
        n143 = Unbundle By Name(w362) -> ("Process Name"=w364:string)
        n144 = Concatenate Strings(w364, " Sequence Start" ("text")) -> (w361:string)
        n145 = call "Write to Log File.vi"("error in"=w365, "text"=w361) -> ()  [unwired: 9 in, 1 out]
      }
      frame "Start Loops" {
        # "Start gets us going"
        # "Message Acquisition and Logging loops to start"
        # "Start - Enable/Disable buttons appropriately for an acquisition that has started, and update status display."
        n146 = Unbundle By Name(w401) -> ("D-O Module Config.Process Name"=w402:string, "D-O Module Config.Settings.Run?"=w396:bool)
        n147 = property class="VI"("Front Panel.Title"=w402) -> ()  [unwired: 2 in, 2 out]
        n148 = call-poly "Enqueue Message.vi"("error in (no error)"=w403, "Message Data"=w402, "Message"="Start", "Message Queue"=w404) -> ("error out"=w399:errorcluster, "dup Message Queue"=w397:refnum<queue>)  [unwired: 6 in]
        n149 = disable-structure shown="Enabled" {
          disable-tunnel: w399 -> [w411 w417]
          disable-tunnel: [w410 w417] -> w398
          disable-tunnel: w397 -> [w409 _]
          disable-tunnel: w396 -> [w408 _]
          frame Disabled {
            n150 = case shown="True" w408 {
              tunnel: w411 -> [w414 w416]
              tunnel: [w413 w416] -> w410
              tunnel: w409 -> [w412 _]
              frame False {
                # "If we are supposed to be paused we pause immediatly"
                n151 = call-poly "Enqueue Message.vi"("error in (no error)"=w414, "Message"="Pause", "Message Queue"=w412) -> ("error out"=w413:errorcluster)  [unwired: 7 in, 1 out]
              }
              frame True {
              }
            }
          }
          frame Enabled {
          }
        }
        n152 = Merge Errors(w398) -> (w407:errorcluster)
      }
      frame "Start Log" {
        # "Message Acquisition and Logging loops to start"
        # "Start - Enable/Disable buttons appropriately for an acquisition that has started, and update status display."
        n153 = Unbundle By Name(w418) -> ("D-O Module Config.Process Name"=w423:string)
        n154 = Build Array(w427) -> (w425:refnum<queue>[])
        n155 = for {
          tunnel: w424 -> [w433]
          tunnel: [w432] -> w426 mode=indexing
          tunnel: w425 -> [w431] mode=indexing
          tunnel: w423 -> [w430]
          n156 = call-poly "Enqueue Message.vi"("error in (no error)"=w433, "Message Data"=w430, "Message"="Start Log", "Message Queue"=w431) -> ("error out"=w432:errorcluster)  [unwired: 6 in, 1 out]
        }
        n157 = property class="VI"("Front Panel.Title"=w423) -> ()  [unwired: 2 in, 2 out]
        n158 = Merge Errors(w426) -> (w422:errorcluster)
        n159 = Unbundle By Name(w418) -> ("Process Name"=w421:string)
        n160 = Concatenate Strings(w421, " Log Started" ("text")) -> (w419:string)
        n161 = call "Write to Log File.vi"("error in"=w422, "text"=w419) -> ()  [unwired: 9 in, 1 out]
      }
      frame "Stop" {
        # "Stop Pauses"
        # "Enable: Start, Exit, Settings\nDisable: Stop"
        # "Stop - Enable/Disable buttons appropriately for an acquisition that has stopped, and update status display."
        n162 = Unbundle By Name(w462) -> ("Trigger Ref"=w453:refnum<vi>, "Stop Ref"=w454:refnum<vi>, "Start Ref"=w457:refnum<vi>, "Exit Ref"=w456:refnum<vi>, "Settings Ref"=w455:refnum<vi>)
        n163 = call-poly "Enqueue Message.vi"("error in (no error)"=w444, "Message"="Broadcast settings", "Message Queue"=w442) -> ("error out"=w443:errorcluster, "dup Message Queue"=w441:refnum<queue>)  [unwired: 7 in]
        n164 = Build Array(w457, w456, w455) -> (w460:refnum<vi>[])
        n165 = Build Array(w453, w454) -> (w459:refnum<vi>[])
        n166 = call-poly "Enqueue Message.vi"("error in (no error)"=w443, "Message Data"="Ready..." ("Ready..."), "Message"="Update Status", "Message Queue"=w441) -> ("error out"=w449:errorcluster)  [unwired: 6 in, 1 out]
        n167 = call "Set Enable State on Multiple Controls.vi"("Enable?"=FALSE, "Controls"=w459) -> ()  [unwired: 10 in]
        n168 = call "Set Enable State on Multiple Controls.vi"("Enable?"=TRUE, "Controls"=w460) -> ()  [unwired: 10 in]
        n169 = call-poly "Enqueue Message.vi"("error in (no error)"=w449, "Message"="Pause", "Message Queue"=w450) -> ("error out"=w447:errorcluster)  [unwired: 7 in, 1 out]
        n170 = case shown="\"Waiting for Exit\"" w451 {
          selector: w451 -> [_ w466]
          tunnel: [UI_State."Waiting for Stop" ("UI State") w466] -> w452
          frame Default {
          }
          frame "Waiting for Exit" {
          }
        }
        n171 = Merge Errors(w447) -> (w439:errorcluster)
        n172 = Bundle By Name(cluster=w446, "State"=State_Enum."Paused") -> (w435:T3)
        n173 = Unbundle By Name(w435) -> ("Process Name"=w438:string)
        n174 = Concatenate Strings(w438, " Stopped" ("text")) -> (w436:string)
        n175 = call "Write to Log File.vi"("error in"=w439, "text"=w436) -> ()  [unwired: 9 in, 1 out]
      }
      frame "Update Status" {
        # "Update Display - Convert the message data to a string to display in the Status indicator."
        n176 = Variant To Data(error in=w477, type="", Variant=w476) -> (data=w470:string, error out=w474:errorcluster)
        "Status" <- w470
        n177 = Unbundle By Name(w473) -> ("Trigger Ref"=w469:refnum<vi>, "Stop Ref"=w472:refnum<vi>)
        n178 = property class="Bool"(reference=w472) -> ("DisabledEnum"=w471:T13)  [unwired: 1 in, 2 out]
        n179 = case shown="\"Enabled\"" w471 {
          tunnel: w470 -> [w481 _]
          tunnel: w469 -> [w482 _]
          frame "Enabled" {
            # "Disable the Force Trigger only while we are logging."
            n180 = Build Array(w482) -> (w483:refnum<vi>[])
            n181 = Not Equal?(x="Logging" ("Logging"), y=w481) -> (x != y?=w479:bool)
            n182 = call "Set Enable State on Multiple Controls.vi"("Enable?"=w479, "Controls"=w483) -> ()  [unwired: 10 in]
          }
          frame "Disabled", Default {
          }
        }
        n183 = Merge Errors(w474) -> (w478:errorcluster)
      }
      frame Default {
        # "'Default' case only runs if there is a message that isn't defined in any of the other cases.  Output a programming error."
        n184 = xnode "Error Ring"("parameter 0"=w486) -> ("error out"=w489:errorcluster)
        n185 = Unbundle By Name(w484) -> ("Process Name"=w488:string)
        n186 = Concatenate Strings(w488, " Invalid Message " ("text"), w486) -> (w485:string)
        n187 = call "Write to Log File.vi"("error in"=w489, "text"=w485) -> ()  [unwired: 9 in, 1 out]
      }
    }
    n188 = Unbundle By Name(w37) -> ()  [unwired: 1 out]
    n189 = call "Error Handler - Message Handling Loop.vi"("error in (no error)"=w51, "Message Queue"=w49) -> ("dup error in"=w50:errorcluster)  [unwired: 8 in, 1 out]
  }
  "Sequence Started" <- w9
  n190 = while {
    tunnel: w28 -> [w508]
    tunnel: [w510] -> w35
    shift-right: [w509] -> w30
    shift-left: w33 -> [w514]
    tunnel: [w507] -> w20
    tunnel: w19 -> [w507]
    tunnel: w14 -> [w506]
    shift-right: [w503] -> _
    shift-left: 500.0 ("Cycle Period") -> [w502]
    stop <- w513 stop-if-true
    # "Event Handling Loop"
    n191 = call "Dequeue Message.vi"("timeout in ms (-1)"=50, "Message Queue"=w506) -> ("error out"=w499:errorcluster, "Message Data"=w504:variant, "Message"=w505:string, "dup Message Queue"=w500:refnum<queue>)  [unwired: 6 in]
    n192 = Flush Queue(queue=w500, error in (no error)=w499) -> ()  [unwired: 3 out]
    n193 = case shown="\"Update\"" w505 {
      tunnel: w504 -> [_ w520]
      tunnel: [w515 w516] -> w503
      tunnel: w502 -> [w515 _]
      frame "False", Default {
      }
      frame "Update" {
        # "Update the display"
        n194 = Variant To Data(type=T14 {"D-O State "=0, "Cycle Period"=0.0} ("FM Display"), Variant=w520) -> (data=w519:T14)  [unwired: 1 in, 1 out]
        n195 = Unbundle By Name(w519) -> ("D-O State"=w518:u16, "Cycle Period"=w516:dbl)
        n196 = case shown="1" w518 {
          frame 0 {
            n197 = local write "Ring"(u16 1 ("Ring")) -> ()
          }
          frame 1 {
            "Ring" <- u16 0 ("Ring")
          }
          frame 2, Default {
            n198 = local write "Ring"(u16 2 ("Ring")) -> ()
          }
        }
      }
    }
    n199 = event "Button Handler" shown="[1] Panel Close?" {
      selector: w514 -> [_ _ _ _ _ _]
      dyn-events: [_ _ _ _ _ _] -> w509
      timeout: w503 -> [_ _ _ _ _ _]
      tunnel: [_ _ _ TRUE ("Discard?") _ _] -> w513
      tunnel: w508 -> [w524 w527 w532 w536 w541 _]
      tunnel: [_ w525 w535 _ w543 _] -> w511
      tunnel: [w524 w526 w531 w536 w542 _] -> w512
      event Timeout {
        n200 = event-data() -> ()  [unwired: 1 in, 1 out]
      }
      event Panel Close? {
        w528 = TRUE  # Priority Message
        n201 = event-data() -> ()  [unwired: 1 in, 1 out]
        n202 = call-poly "Enqueue Message.vi"("Priority Message? (F)"=w528, "Message"="Confirm Quit", "Message Queue"=w527) -> ("error out"=w525:errorcluster, "dup Message Queue"=w526:refnum<queue>)  [unwired: 7 in]
        n203 = event-data("Discard?"=TRUE) -> ()  [unwired: 1 in, 1 out]
      }
      event "Exit": Value Change {
        w533 = TRUE  # Priority Message
        # "The UI Message Loop handles sending the Exit message to other loops."
        n204 = event-data() -> ()  [unwired: 1 in, 1 out]
        n205 = call-poly "Enqueue Message.vi"("Priority Message? (F)"=w533, "Message"="Exit", "Message Queue"=w532) -> ("error out"=w535:errorcluster, "dup Message Queue"=w531:refnum<queue>)  [unwired: 7 in]
      }
      event User Event {
        # "The Message Handling Loop processed an \"Exit\" message, which fired this event to stop the Event Handling Loop."
        n206 = event-data() -> ()  [unwired: 1 in, 1 out]
        n207 = local write "Status"("Exit" ("Exit String")) -> ()
      }
      event "Settings Button": Mouse Down {
        n208 = event-data() -> ("PlatMods"=w540:T15)  [unwired: 1 in]
        n209 = Unbundle By Name(w540) -> ("Ctrl"=w539:bool)
        n210 = case shown="True" w539 {
          tunnel: [w547 w548] -> w543
          tunnel: [w546 w549] -> w542
          tunnel: w541 -> [w545 w549]
          frame False {
            n211 = call-poly "Enqueue Message.vi"("Message"="Launch Settings Dialog", "Message Queue"=w545) -> ("error out"=w547:errorcluster, "dup Message Queue"=w546:refnum<queue>)  [unwired: 8 in]
          }
          frame True {
            n212 = property class="VI"("BDWin.Open"=TRUE ("Block Diagram Window:Open")) -> (error out=w548:errorcluster)  [unwired: 2 in, 1 out]
          }
        }
      }
      event Key Down {
        n213 = event-data() -> ("ScanCode"=→"ScanCode":i16)  [unwired: 1 in]
      }
    }
    n214 = call "Error Handler - Event Handling Loop.vi"("error in (no error)"=w511, "Message Queue"=w512) -> ("dup error in"=w510:errorcluster)  [unwired: 8 in, 1 out]
  }
  n215 = call "Main Loop.vi"("error in (no error)"=w3, "Chart Notifier"=w21, "Message Queues"=w12) -> ("error out"=w22:errorcluster)  [unwired: 8 in]
  n216 = Unregister For Events(event registration refnum=w30, error in=w35) -> (error out=w31:errorcluster)
  n217 = Close Reference(reference=w20) -> ()  [unwired: 1 in, 1 out]
  n218 = Merge Errors(w31, w36, w3, w22) -> (w34:errorcluster)
  n219 = call "Destroy User Event - Stop.vi"("error in (no error)"=w34, "User Event - Stop"=w32) -> ()  [unwired: 9 in, 1 out]
